vi "BSCAN_DEMO01_GPIO_writeRead.vi"() -> ()   [LabVIEW 2017]
uses:
  Saldigi_protocol_library.lvlibp
panel:
  out "port state in":bool
  out "PORT state out":bool
  in  "duplicate data":T1(ring)
  in  "Version":enum16{"BSCAN V1", "BSCAN V2"}(ring)=enum."BSCAN V2"
  out "BSCAN Code+BUS dt (s)":dbl=0.005799500038847327
  in  "CHAINn/TARGETn/PORTn in":string(combo)="chain0/xc7z020_clg400/IO_P18"
  in  "stop":bool
  in  "milliseconds to wait":u32(knob)=116 scale=0.0..500.0
  out "error out":errorcluster
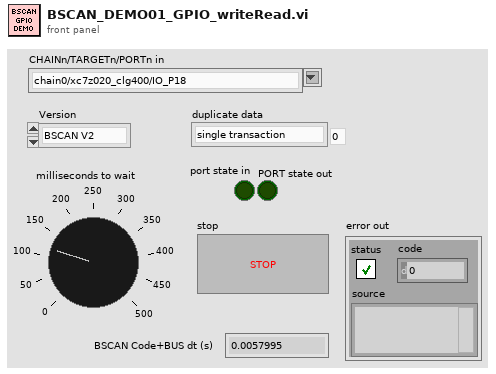
[diagram p1: front panel]
types:
  T1 = enum16{"single transaction", "double transaction"}
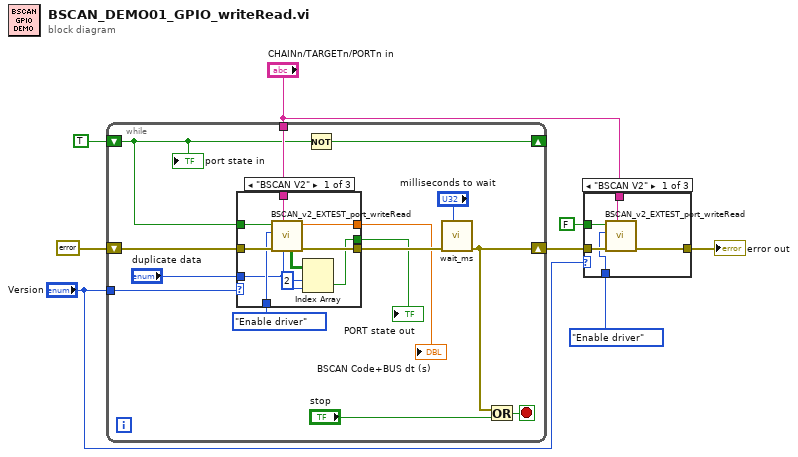
[diagram p0: block diagram]
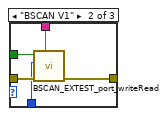
[diagram p2: hidden frame]
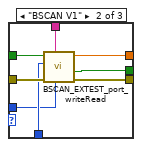
[diagram p4: hidden frame]
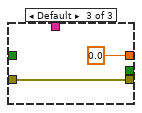
[diagram p5: hidden frame]
diagram:
  n1 = while {
    shift-right: [w13] -> w6
    shift-left: errorcluster {"status"=FALSE, "code"=0, "source"=""} ("error in") -> [w22]
    tunnel: "CHAINn/TARGETn/PORTn in" -> [w20]
    shift-right: [w17] -> _
    shift-left: TRUE ("port state in") -> [w18]
    tunnel: "Version" -> [w12]
    stop <- w15 stop-if-true
    n2 = case shown="\"BSCAN V2\"" w12 {
      tunnel: w22 -> [w30 w40 w42]
      tunnel: [w29 w39 w42] -> w21
      tunnel: w20 -> [w32 w38 _]
      tunnel: w18 -> [w31 w37 _]
      tunnel: [w28 w36 0.0 ("dt")] -> w16
      tunnel: enum16{"Enable driver", "Disable driver"}."Enable driver" ("port driver state in") -> [w27 w35 _]
      tunnel: [w23 w34 _] -> w9
      tunnel: "duplicate data" -> [w25 w33 _]
      frame "BSCAN V2" {
        n3 = call "BSCAN_v2_EXTEST_port_writeRead.vi"("duplicate data"=w25, "CHAINn/TARGETn/PORTn in"=w32, "error in"=w30, "port driver state in"=w27, "port state in"=w31) -> ("error out"=w29:errorcluster, "dt"=w28:dbl, "elements out"=w26:bool[][])  [unwired: 4 in]
        n4 = Index Array(array=w26, index (row)=2 ("disabled index (row)"), index (col)=w25) -> (element=w23:bool)
      }
      frame "BSCAN V1" {
        n5 = call "BSCAN_EXTEST_port_writeRead.vi"("duplicate data"=w33, "CHAINn/TARGETn/PORTn in"=w38, "error in"=w40, "port driver state in"=w35, "port state in"=w37) -> ("error out"=w39:errorcluster, "PORT state out"=w34:bool, "dt"=w36:dbl)  [unwired: 4 in]
      }
      frame Default {
      }
    }
    "BSCAN Code+BUS dt (s)" <- w16
    "PORT state out" <- w9
    n6 = Not(x=w18) -> (.not. x?=w17:bool)
    n7 = call "wait_ms.vi"("milliseconds to wait"="milliseconds to wait", "error in"=w21) -> ("error out"=w13:errorcluster)  [unwired: 9 in]
    n8 = Or(x=w13, y="stop") -> (x .or. y?=w15:bool)
    "port state in" <- w18
  }
  n9 = case shown="\"BSCAN V2\"" "Version" {
    tunnel: w6 -> [w47 w52 w53]
    tunnel: enum16{"Enable driver", "Disable driver"}."Enable driver" ("port driver state in") -> [w43 w51 _]
    tunnel: FALSE ("port state in") -> [w45 w50 _]
    tunnel: "CHAINn/TARGETn/PORTn in" -> [w44 w49 _]
    tunnel: [w46 w48 w53] -> w2
    frame "BSCAN V2" {
      n10 = call "BSCAN_v2_EXTEST_port_writeRead.vi"("CHAINn/TARGETn/PORTn in"=w44, "error in"=w47, "port driver state in"=w43, "port state in"=w45) -> ("error out"=w46:errorcluster)  [unwired: 5 in, 2 out]
    }
    frame "BSCAN V1" {
      n11 = call "BSCAN_EXTEST_port_writeRead.vi"("CHAINn/TARGETn/PORTn in"=w49, "error in"=w52, "port driver state in"=w51, "port state in"=w50) -> ("error out"=w48:errorcluster)  [unwired: 5 in, 2 out]
    }
    frame Default {
    }
  }
  "error out" <- w2
